vi "DAQ_Digital Clk Gen Initialize.vi"(0 "Physical Channel (Counter)":tag, 2 "Output Terminal":tag, 11 "error in":errorcluster) -> (4 "DAQmx Task Out":refnum<k21>, 15 "error out":errorcluster)   [LabVIEW 2021, in "DAQ_Digital Clock Generation.lvlib"]
doc: "Initialize counter output channel and obtains a DAQmx task. Get Physical channel of counter and output terminal to generate.\n\nNote: Multiple counters cannot be initialized in the same task. Use a separate task for each counter.\nGlobal Channel and Frequency Generator(FreqOut) is not supported for this library"
uses:
  DAQ_Digital Clock Generation.lvlib
  <vilib>/DAQmx/create/channels.llb/DAQmx Create Channel (CO-Pulse Generation-Frequency).vi
  <resource>/objmgr/daqmx.rc
panel:
  # "Inputs"
  # "Outputs"
  # "Overview:\nThis VI initializes Counter of TestScale DIO Module and provides the DAQmx Task Out\n\nHardware Requirement: A compatible PXI, PCIe, USB, cDAQ or Testscale device\n\nSoftware Requirement: NI DAQmx 2022 Q4 or later\n\nInstructions:\n1. Enter physical channel of counter to use for Digital clock generation in Physical Channels control.\n2. Enter Output Terminal on which the signal to be measured. Refer Help for more details on the default terminals of each counters. User can configure different PFI lines as well. \n3. Get the Digital Clock Generation task from DAQmx Task Out\n\nNotes: User can use the DAQmx Task on other VIs to configure and initiate Digital Clock Generation.\nMultiple counters cannot be initialized in the same task. Use a separate task for each counter."
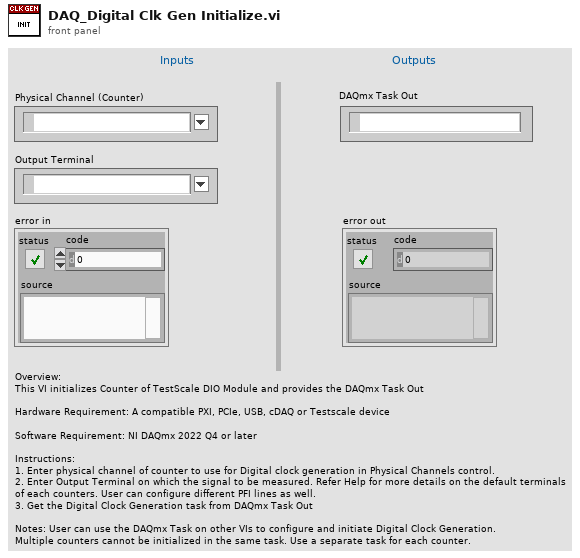
[diagram p1: front panel]
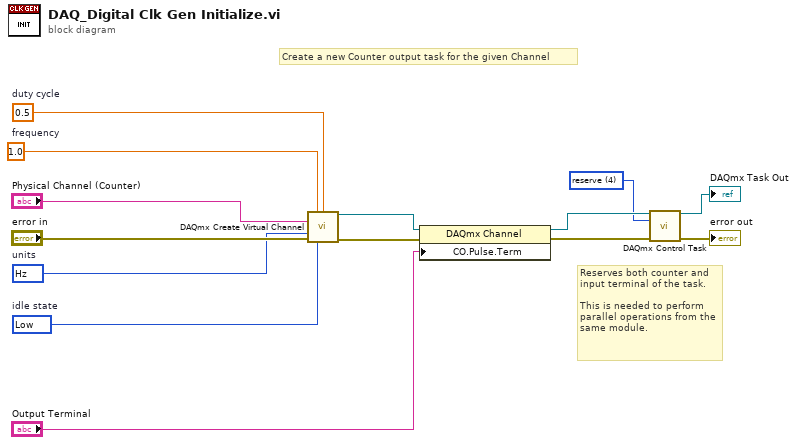
[diagram p0: block diagram]
diagram:
  w1 = 0.5  # duty cycle
  w2 = 1.0  # frequency
  w3 = 10373 items=["Hz"=10373]  # units
  w4 = 10214 items=["High"=10192, "Low"=10214]  # idle state
  w5 = 4 items=["verify"=2, "reserve"=4, "commit"=3, "unreserve"=5, "abort"=6] ("action")
  # "Create a new Counter output task for the given Channel"
  # "Reserves both counter and input terminal of the task.\n\nThis is needed to perform parallel operations from the same module."
  n1 = call-poly <vilib>:"DAQmx Create Virtual Channel.vi"("frequency"=w2, "duty cycle"=w1, "counter"="Physical Channel (Counter)", "units"=w3, "error in"="error in", "idle state"=w4) -> ("task out"=w10:refnum<k21>, "error out"=w13:errorcluster)  [unwired: 8 in]
  n2 = property class="DAQmx Channel"(reference=w10, error in=w13, "CO.Pulse.Term"="Output Terminal") -> (reference out=w7:refnum<k21>, error out=w11:errorcluster)
  n3 = call <vilib>:"DAQmx Control Task.vi"("task/channels in"=w7, "action"=w5, "error in"=w11) -> ("task out"=→"DAQmx Task Out":refnum<k21>, "error out"=→"error out":errorcluster)  [unwired: 11 in]
